vi "simulador.vi"(8 "error in (no error)":errorcluster, 10 "valor":dbl=0.75 format="%#_13g", 11 "Keithley2002 in":refnum<class "Keithley2002.lvclass">) -> (0 "error out":errorcluster, 2 "medicion":dbl, 3 "Keithley2002 out":refnum<class "Keithley2002.lvclass">)   [LabVIEW 2019, in "Keithley2002.lvclass"]
uses:
  Keithley2002.lvclass
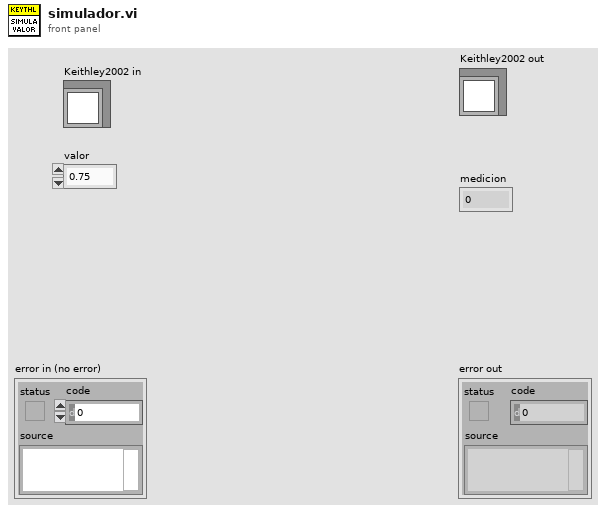
[diagram p1: front panel]
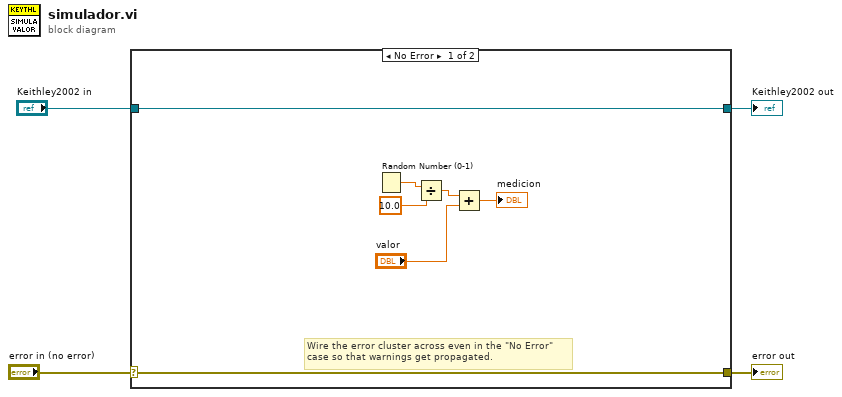
[diagram p0: block diagram]
diagram:
  n1 = case shown="No Error" "error in (no error)" {
    selector: "error in (no error)" -> [w10 w13]
    tunnel: [w10 w13] -> w3
    tunnel: [w11 w12] -> w1
    tunnel: "Keithley2002 in" -> [w11 w12]
    frame No Error {
      # "Wire the error cluster across even in the \"No Error\"\ncase so that warnings get propagated."
      n2 = Random Number (0-1)() -> (number: 0 to 1=w8:dbl)
      n3 = Divide(x=w8, y=10.0) -> (x/y=w6:dbl)
      n4 = Add(x=w6, y="valor") -> (x+y=→"medicion":dbl)
    }
    frame Error {
    }
  }
  "error out" <- w3
  "Keithley2002 out" <- w1
